vi "DebugCommunication.vi"() -> ()   [LabVIEW 2017, in "Server.lvlib" / "Message Queue.lvlib"]
doc: "This VI reads the \"TrackerQueue\" and displays the contained Data (all messages sent in the Host-Application) in different ways."
uses:
  Message Queue.lvlib
  Debug_TrackerData.ctl
  MessageCluster.ctl
panel:
  in  "Blank Button":bool
  in  "Queues":i32[](listbox)
  in  "Messages":i32[](listbox)
  out "Table":string[][](table)
  in  "Stop Button":bool
  # "Instruction:\nStart this Tracker before or while the Host-VI is running. If you want to see Initialization-Messages, you have to start it before you run the Main VI!\n\nIt will display all Messages in all Queues by default. You can use the left Filter-Lists to only display specific Messages or Messages in specific Queues. You can multiselect Listitems by Ctrl+Click."
  # "Hover over the Data-Column-Fields or increase the Row-Height to display the full data in XML-Notation.\n\nThe Call-Chain shows from which VI the Message was sent. Sadly It can't display the Loop where it comes from, but at least you see if it came from a SubVI or the Main VI."
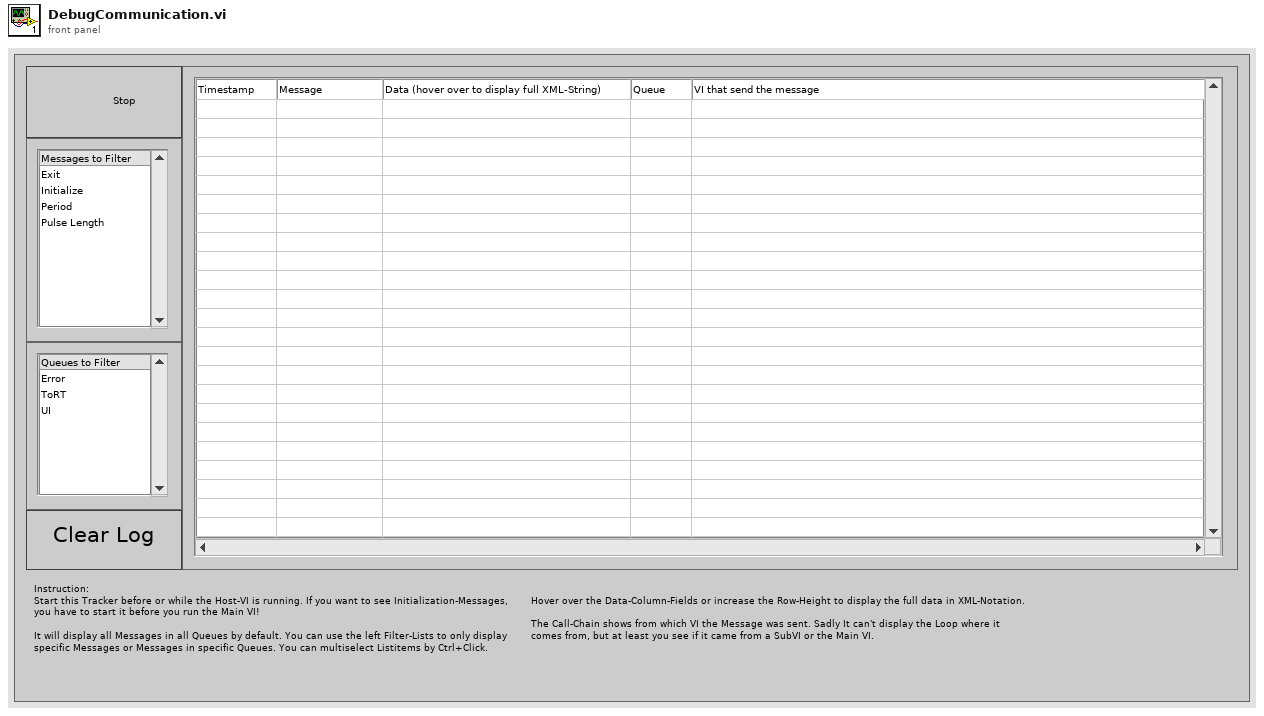
[diagram p1: front panel]
types:
  T1 = typedef "Server.lvlib/Message Queue.lvlib/Debug_TrackerData.ctl" = cluster{"Time Stamp":timestamp, "Message Cluster":T2, "CallChain":string[], "QueueName":string}
  T2 = typedef "Server.lvlib/Message Queue.lvlib/MessageCluster.ctl" = cluster{"Message":string, "Message Data":variant}
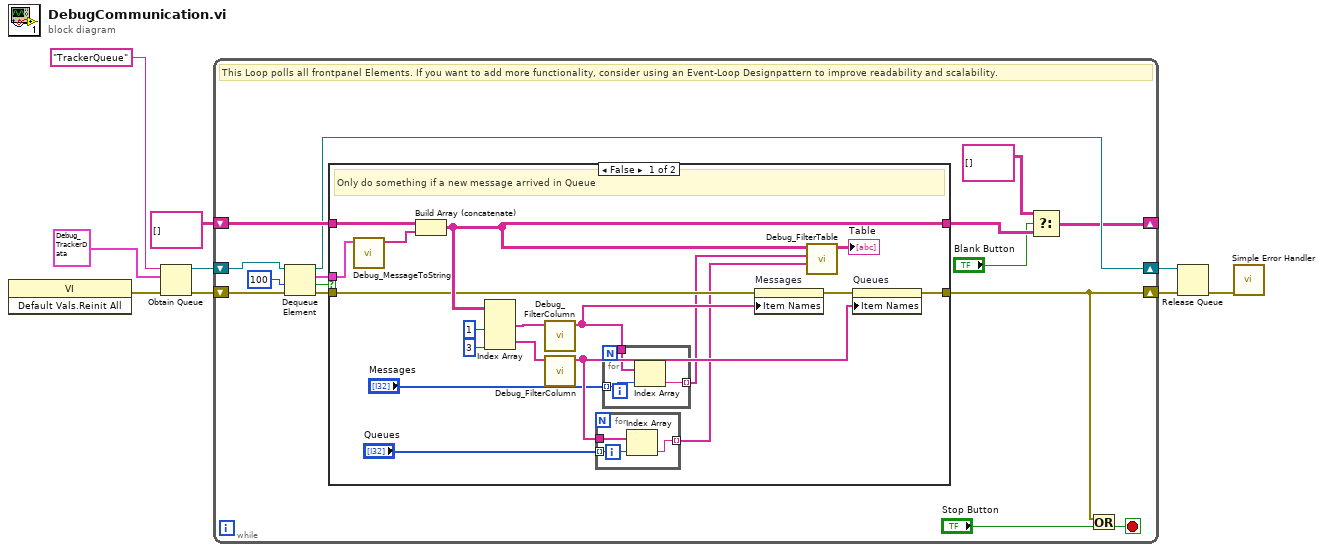
[diagram p0: block diagram]
diagram:
  n1 = invoke class="VI" method="Default Vals.Reinit All"() -> (error out=w6:errorcluster)  [unwired: 3 in, 2 out]
  n2 = Obtain Queue(name (unnamed)="TrackerQueue", element data type=T1 {"Time Stamp"=timestamp(0 s since 1904-01-01), "Message Cluster"={"Message"="", "Message Data"=variant}, "CallChain"=[], "QueueName"=""} ("TrackerData"), error in (no error)=w6) -> (queue out=w8:refnum<queue>, error out=w7:errorcluster)  [unwired: 2 in, 1 out]
  n3 = while {
    shift-right: [w13] -> _
    shift-left: string[][] [] -> [w18]
    shift-right: [w14] -> w4
    shift-left: w7 -> [w23]
    shift-right: [w17] -> w3
    shift-left: w8 -> [w24]
    stop <- w16 stop-if-true
    # "This Loop polls all frontpanel Elements. If you want to add more functionality, consider using an Event-Loop Designpattern to improve readability and scalability."
    n4 = Dequeue Element(queue=w24, timeout in ms (-1)=100, error in (no error)=w23) -> (queue out=w17:refnum<queue>, element=w21:T1, timed out?=w19:bool, error out=w15:errorcluster)
    n5 = case shown="False" w19 {
      tunnel: w21 -> [w42 _]
      tunnel: [w39 w50] -> w12
      tunnel: w18 -> [w41 w50]
      tunnel: w15 -> [w34 w49]
      tunnel: [w32 w49] -> w14
      frame False {
        # "Only do something if a new message arrived in Queue"
        n6 = call "Debug_MessageToString.vi"("TrackerData"=w42) -> ("Array"=w40:string[])  [unwired: 10 in]
        n7 = Build Array (concatenate)(w41, w40) -> (w39:string[][])
        n8 = Index Array(array=w39, index (col) #1=1 ("disabled index (col)"), index (col) #2=3 ("index (col)")) -> (element #1=w36:string[], element #2=w35:string[])  [unwired: 2 in]
        n9 = call "Debug_FilterColumn.vi"("Array in"=w36) -> ("Array out"=w30:string[])  [unwired: 10 in]
        n10 = call "Debug_FilterColumn.vi"("Array in"=w35) -> ("Array out"=w29:string[])  [unwired: 10 in]
        n11 = for {
          tunnel: w29 -> [w45]
          tunnel: "Queues" -> [w44] mode=indexing
          tunnel: [w43] -> w25 mode=indexing
          n12 = Index Array(array=w45, index=w44) -> (element=w43:string)
        }
        n13 = for {
          tunnel: w30 -> [w48]
          tunnel: "Messages" -> [w47] mode=indexing
          tunnel: [w46] -> w26 mode=indexing
          n14 = Index Array(array=w48, index=w47) -> (element=w46:string)
        }
        n15 = property on="Messages" class="LstBox (strict)"(error in=w34, "Item Names"=w30) -> (error out=w33:errorcluster)  [unwired: 1 in, 1 out]
        n16 = call "Debug_FilterTable.vi"("QueuesToDisplay"=w25, "MessagesToDisplay"=w26, "Array in"=w39) -> ("Array out"=→"Table":string[][])  [unwired: 8 in]
        n17 = property on="Queues" class="LstBox (strict)"(error in=w33, "Item Names"=w29) -> (error out=w32:errorcluster)  [unwired: 1 in, 1 out]
      }
      frame True {
      }
    }
    n18 = Select(t=string[][] [], s="Blank Button", f=w12) -> (s? t:f=w13:string[][])
    n19 = Or(x=w14, y="Stop Button") -> (x .or. y?=w16:bool)
  }
  n20 = Release Queue(queue=w3, error in (no error)=w4) -> (error out=w2:errorcluster)  [unwired: 1 in, 2 out]
  n21 = call <vilib>:"Simple Error Handler.vi"("error in (no error)"=w2) -> ()  [unwired: 4 in, 5 out]
